vi "Check KeyUp.vi"(9 "Shift":bool, 11 "ScanCode":i16) -> (2 "Task":string)   [LabVIEW 2022 SP3]
uses:
  Mic/Mic_Global.vi
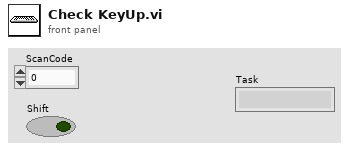
[diagram p1: front panel]
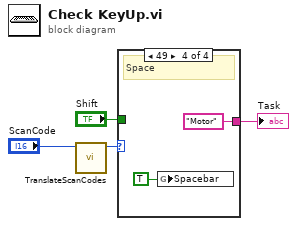
[diagram p0: block diagram]
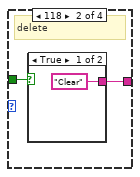
[diagram p3: hidden frame]
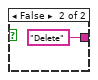
[diagram p4: hidden frame]
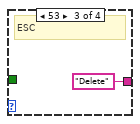
[diagram p5: hidden frame]
diagram:
  n1 = call "TranslateScanCodes.vi"("ScanCode in"="ScanCode") -> ("ScanCode out"=w3:i16)  [unwired: 10 in]
  n2 = case shown="49" w3 {
    tunnel: "Shift" -> [_ w6 _ _]
    tunnel: [_ w5 "Delete" "Motor"] -> w1
    frame 0, Default {
    }
    frame 118 {
      # "delete"
      n3 = case shown="True" w6 {
        tunnel: ["Clear" "Delete"] -> w5
        frame True {
        }
        frame False {
        }
      }
    }
    frame 53 {
      # "ESC"
    }
    frame 49 {
      # "Space"
      n4 = global write "Mic_Global.vi" "Spacebar"(TRUE ("Spacebar")) -> ()
    }
  }
  "Task" <- w1
